vi "begin5RobotsNormalGamePlay.vi"(8 "error in (no error)":errorcluster, 9 "Game in":refnum<class "Game.lvclass">, 10 "AnyPlayChosen?":bool, 11 "5RobotsNormalGamePlay in":refnum<class "5RobotsNormalGamePlay.lvclass">) -> (0 "error out":errorcluster, 1 "Game out":refnum<class "Game.lvclass">, 2 "begin?":bool, 3 "5RobotsNormalGamePlay out":refnum<class "5RobotsNormalGamePlay.lvclass">)   [LabVIEW 2020, in "5RobotsNormalGamePlay.lvclass"]
uses:
  5RobotsNormalGamePlay.lvclass
  Game_class/Game.lvclass
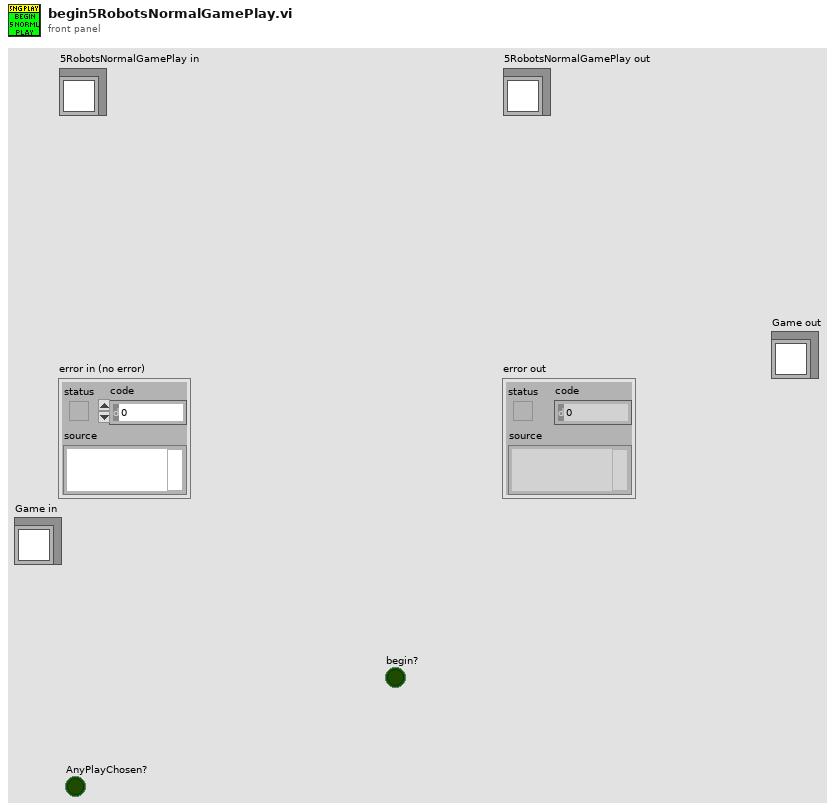
[diagram p1: front panel]
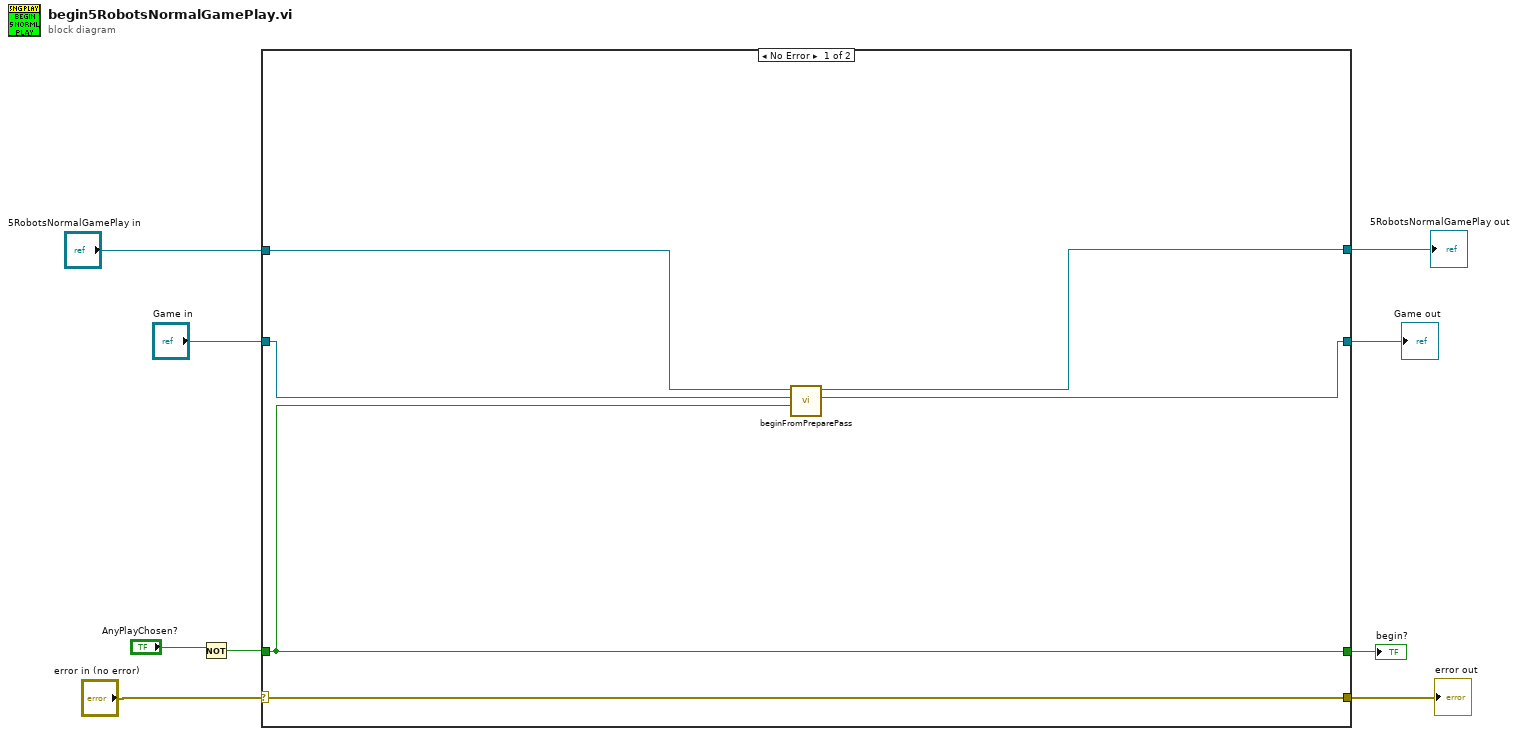
[diagram p0: block diagram]
diagram:
  n1 = Not(x="AnyPlayChosen?") -> (.not. x?=w8:bool)
  n2 = case shown="No Error" "error in (no error)" {
    selector: "error in (no error)" -> [w15 w18]
    tunnel: [w15 w18] -> w5
    tunnel: [w10 w17] -> w4
    tunnel: "5RobotsNormalGamePlay in" -> [w11 w17]
    tunnel: w8 -> [w14 _]
    tunnel: [w14 _] -> w9
    tunnel: [w13 w16] -> w2
    tunnel: "Game in" -> [w12 w16]
    frame No Error {
      n3 = call "beginFromPreparePass.vi"("begin?"=w14, "Game in"=w12, "5RobotsNormalGamePlay in"=w11) -> ("Game out"=w13:refnum<class "Game.lvclass">, "5RobotsNormalGamePlay out"=w10:refnum<class "5RobotsNormalGamePlay.lvclass">)  [unwired: 7 in]
    }
    frame Error {
    }
  }
  "error out" <- w5
  "5RobotsNormalGamePlay out" <- w4
  "begin?" <- w9
  "Game out" <- w2
